vi "formating.vi"() -> ()   [LabVIEW 2020]
uses:
  <vilib>/Utility/config.llb/NI_LVConfig.lvlib
  common/features/CF-common_features.lvlib
panel:
  out "resulting string 3":string
  out "resulting string 2":string
  out "resulting string":string
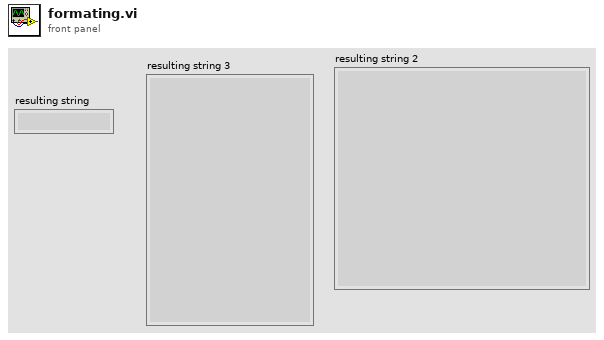
[diagram p1: front panel]
types:
  T1 = enum16{"open", "replace", "create", "open or create", "replace or create", "replace or create with confirmation"}
  T2 = cluster{"signal info":cluster{"Start":dbl, "Stop":dbl, "Points":u32}, "S-Parameter":string}
  T3 = cluster{"software info":string, "date":string, "file content info":string, "signal name":string, "info":string, "signals":string, "sdsad":string}
  T4 = cluster{"software info":string, "date":timestamp, "comment":string, "device":string}
  T5 = typedef "NI_LVConfig.lvlib/Config Data RefNum.ctl" = refnum<k1>
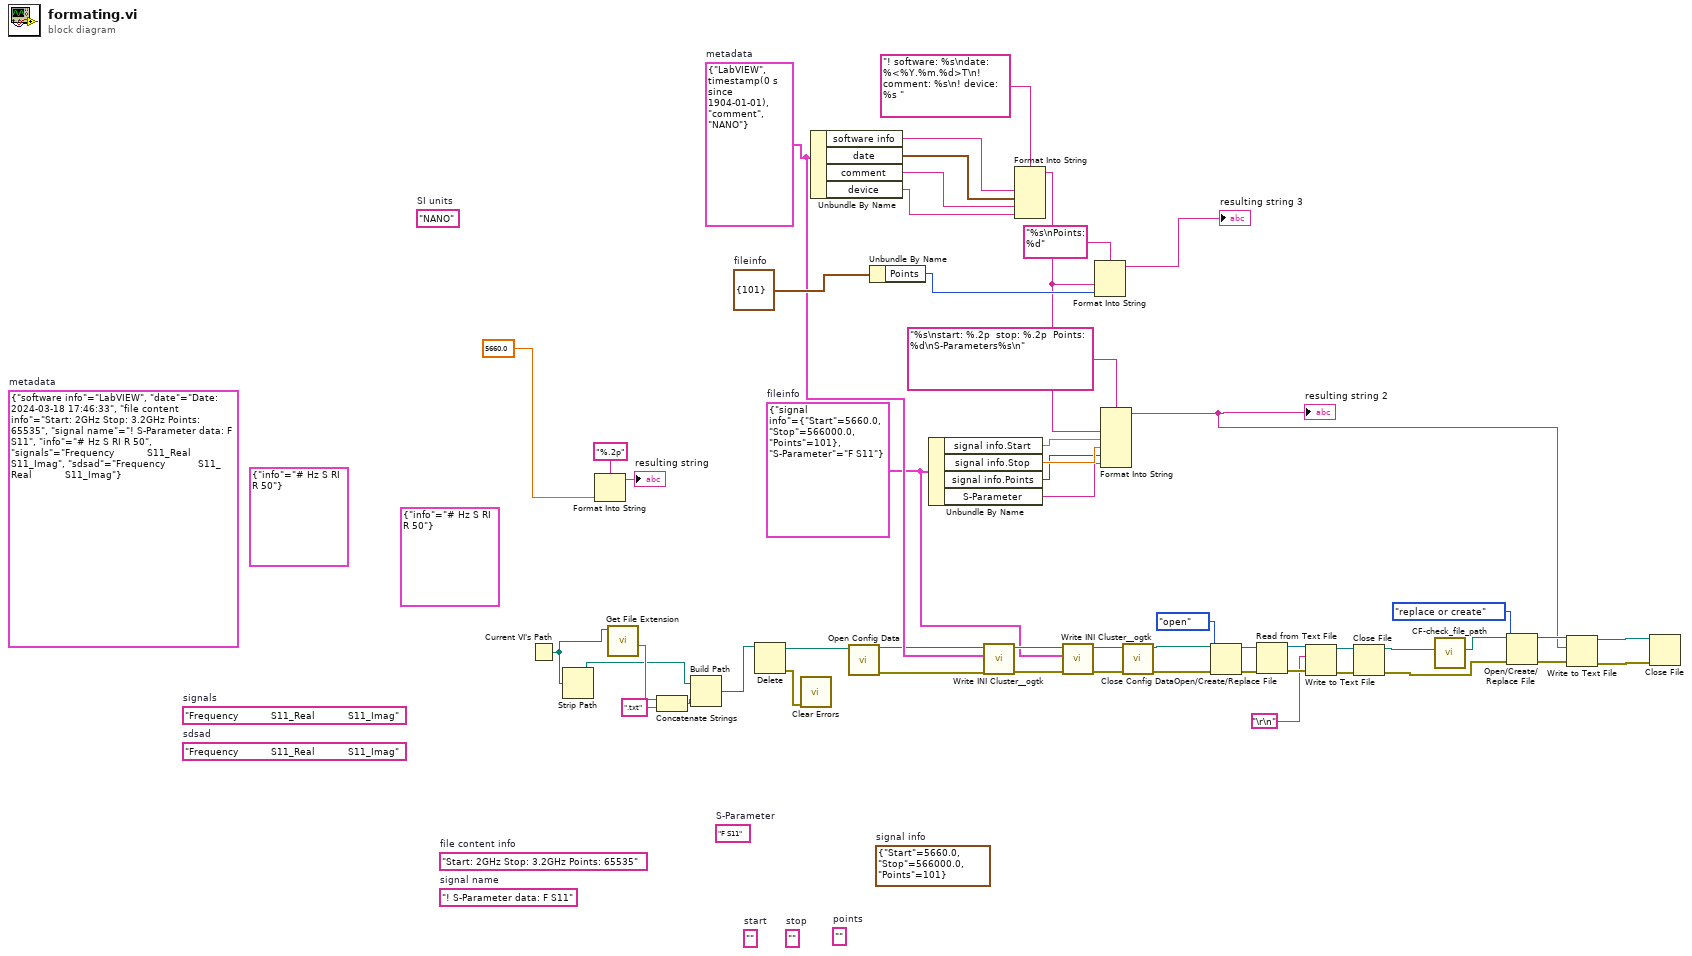
[diagram p0: block diagram]
diagram:
  (unwired) "NANO"  # SI units
  (unwired) "F S11"  # S-Parameter
  (unwired) cluster{"Start":dbl, "Stop":dbl, "Points":u32} {"Start"=5660.0, "Stop"=566000.0, "Points"=101}  # signal info
  w44 = cluster{"Points":u32} {"Points"=101}  # fileinfo
  w32 = T2 {"signal info"={"Start"=5660.0, "Stop"=566000.0, "Points"=101}, "S-Parameter"="F S11"}  # fileinfo
  (unwired) cluster{"info":string} {"info"="# Hz S RI R 50"}
  (unwired) ""  # points
  (unwired) ""  # stop
  (unwired) ""  # start
  (unwired) cluster{"info":string} {"info"="# Hz S RI R 50"}
  (unwired) "Frequency           S11_Real           S11_Imag"  # sdsad
  (unwired) "Frequency           S11_Real           S11_Imag"  # signals
  (unwired) "! S-Parameter data: F S11"  # signal name
  (unwired) "Start: 2GHz Stop: 3.2GHz Points: 65535"  # file content info
  (unwired) T3 {"software info"="LabVIEW", "date"="Date: 2024-03-18 17:46:33", "file content info"="Start: 2GHz Stop: 3.2GHz Points: 65535", "signal name"="! S-Parameter data: F S11", "info"="# Hz S RI R 50", "signals"="Frequency           S11_Real           S11_Imag", "sdsad"="Frequency           S11_Real           S11_Imag"}  # metadata
  w33 = T4 {"software info"="LabVIEW", "date"=timestamp(0 s since 1904-01-01), "comment"="comment", "device"="NANO"}  # metadata
  n1 = Current VI's Path() -> (path=w16:path)
  n2 = Strip Path(path=w16) -> (stripped path=w14:path)  [unwired: 1 out]
  n3 = Format Into String(format string="%.2p", 5660.0 ("number")) -> (resulting string=→"resulting string":string)  [unwired: 2 in, 1 out]
  n4 = call <vilib>:"Get File Extension.vi"("file"=w16) -> ("filename without extension"=w15:string)  [unwired: 6 in, 4 out]
  n5 = Concatenate Strings(w15, ".txt" ("string")) -> (w13:string)
  n6 = Build Path(base path=w14, name or relative path=w13) -> (appended path=w11:path)
  n7 = Delete(path (use dialog)=w11) -> (deleted path=w27:path, error out=w1:errorcluster)  [unwired: 4 in, 1 out]
  n8 = call <vilib>:"Clear Errors.vi"("error in (no error)"=w1) -> ()  [unwired: 5 in, 2 out]
  n9 = Unbundle By Name(w33) -> ("software info"=w48:string, "date"=w49:timestamp, "comment"=w47:string, "device"=w46:string)
  n10 = call <vilib>:"Open Config Data.vi"("configuration file path"=w27) -> ("error out"=w29:errorcluster, "refnum"=w30:T5)  [unwired: 8 in, 1 out]
  n11 = Unbundle By Name(w44) -> ("Points"=w43:u32)
  n12 = Unbundle By Name(w32) -> ("signal info.Start"=w40:dbl, "signal info.Stop"=w39:dbl, "signal info.Points"=w38:u32, "S-Parameter"=w37:string)
  n13 = call <userlib>:"Write INI Cluster__ogtk.vi"("error in (no error)"=w29, "INI Fomatted Cluster"=w33, "refnum"=w30) -> ("error out"=w34:errorcluster, "dup refnum"=w35:T5)  [unwired: 7 in]
  n14 = Format Into String(format string="! software: %s\ndate: %<%Y.%m.%d>T\n! comment: %s\n! device: %s ", w48, w49, w47, w46) -> (resulting string=w41:string)  [unwired: 2 in, 1 out]
  n15 = call <userlib>:"Write INI Cluster__ogtk.vi"("error in (no error)"=w34, "INI Fomatted Cluster"=w32, "refnum"=w35) -> ("error out"=w28:errorcluster, "dup refnum"=w31:T5)  [unwired: 7 in]
  n16 = Format Into String(format string="%s\nPoints: %d", w41, w43) -> (resulting string=→"resulting string 3":string)  [unwired: 2 in, 1 out]
  n17 = Format Into String(format string="%s\nstart: %.2p  stop: %.2p  Points: %d\nS-Parameters%s\n", w41, w40, w39, w38, w37) -> (resulting string=w3:string)  [unwired: 2 in, 1 out]
  "resulting string 2" <- w3
  n18 = call <vilib>:"Close Config Data.vi"("error in (no error)"=w28, "refnum"=w31) -> ("error out"=w18:errorcluster, "file path"=w19:path)  [unwired: 8 in]
  n19 = Open/Create/Replace File(file path (use dialog)=w19, error in=w18, operation (0:open)=T1."open") -> (refnum out=w24:refnum<file>, error out=w23:errorcluster)  [unwired: 3 in, 1 out]
  n20 = Read from Text File(file (use dialog)=w24, error in=w23) -> (refnum out=w25:refnum<file>, error out=w26:errorcluster)  [unwired: 2 in, 2 out]
  n21 = Write to Text File(file (use dialog)=w25, text="\r\n", error in=w26) -> (refnum out=w21:refnum<file>, error out=w20:errorcluster)  [unwired: 1 in, 1 out]
  n22 = Close File(refnum=w21, error in=w20) -> (path=w10:path, error out=w2:errorcluster)
  n23 = call "CF-check_file_path.vi"("File Path"=w10) -> ("File Path out"=w6:path)  [unwired: 10 in]
  n24 = Open/Create/Replace File(file path (use dialog)=w6, error in=w2, operation (0:open)=T1."replace or create") -> (refnum out=w5:refnum<file>, error out=w4:errorcluster)  [unwired: 3 in, 1 out]
  n25 = Write to Text File(file (use dialog)=w5, text=w3, error in=w4) -> (refnum out=w8:refnum<file>, error out=w9:errorcluster)  [unwired: 1 in, 1 out]
  n26 = Close File(refnum=w8, error in=w9) -> ()  [unwired: 2 out]
